vi "High Temp.vi"(1 "Temperature (in *C)":dbl) -> (0 "High Temp":bool)   [LabVIEW 2019]
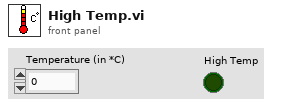
[diagram p1: front panel]
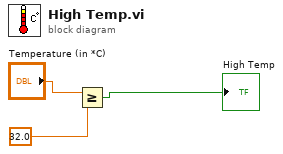
[diagram p0: block diagram]
diagram:
  n1 = Greater Or Equal?(x="Temperature (in *C)", y=32.0) -> (x >= y?=→"High Temp":bool)
